vi "test_ClientFGV_GetClientErrors_ClientNotCreated.vi"(8 "error in":errorcluster) -> (0 "error out":errorcluster, 2 "result":string, 3 "pass":bool)   [LabVIEW 2020, in "MeasurementServerTests.lvlib" / "gRPC Utilities Tests.lvlib"]
uses:
  gRPC Utilities Tests.lvlib
  Runtime/MeasurementLink gRPC Utilities/TypeDefs/Client Pool FGV Action.ctl
  Fake Client Action.ctl
  Runtime/MeasurementLink gRPC Utilities/MeasurementLink gRPC Utilities.lvlib
  MeasurementServerTests.lvlib
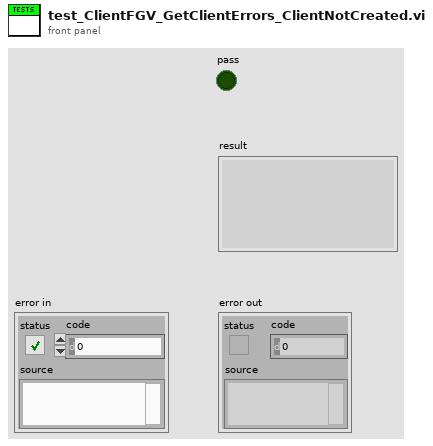
[diagram p1: front panel]
types:
  T1 = typedef "MeasurementServerTests.lvlib/gRPC Utilities Tests.lvlib/Fake Client Action.ctl" = enum16{"Generate New Id", "Reset", "Error on Next Call"}
  T2 = typedef "MeasurementLink gRPC Utilities.lvlib/Client Pool FGV Action.ctl" = enum16{"Get Client", "Recreate Client"}
  T3 = typedef "grpc-lvsupport-release.lvlib/grpcId.ctl" = u64
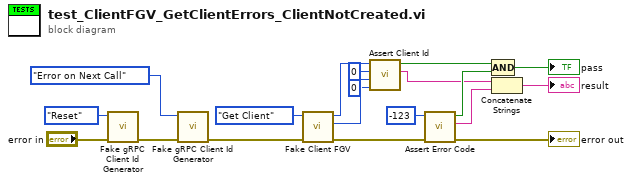
[diagram p0: block diagram]
diagram:
  n1 = call "Fake gRPC Client Id Generator.vi"("error in"="error in", "action"=Fake_Client_Action."Reset") -> ("error out"=w14:errorcluster)  [unwired: 8 in, 1 out]
  n2 = call "Fake gRPC Client Id Generator.vi"("error in"=w14, "action"=Fake_Client_Action."Error on Next Call") -> ("error out"=w15:errorcluster)  [unwired: 8 in, 1 out]
  n3 = call "Fake Client FGV.vi"("error in"=w15, "action"=Client_Pool_FGV_Action."Get Client") -> ("error out"=w12:errorcluster, "unique id out"=w7:u64, "grpc client id"=w8:T3)  [unwired: 7 in]
  n4 = call "Assert Client Id.vi"("expected unique id"=u64 0, "actual unique id"=w7, "expected client id"=u64 0, "actual client id"=w8) -> ("result"=w3:string, "pass"=w4:bool)  [unwired: 6 in]
  n5 = call "Assert Error Code.vi"("error in"=w12, "expected error code"=-123) -> ("error out"=→"error out":errorcluster, "details"=w1:string, "error code match?"=w9:bool)  [unwired: 7 in]
  n6 = Compound Arithmetic op=AND(w4, w9) -> (→"pass":bool)
  n7 = Concatenate Strings(w3, w1) -> (→"result":string)
